vi "Actual Record Length.vi"(8 "error in (no error)":errorcluster, 11 "CS++Scope":refnum<class "CS++Scope.lvclass">) -> (0 "error out":errorcluster, 2 "actual record length":i32 caption="actual record length (samples)", 3 "CS++Scope out":refnum<class "CS++Scope.lvclass">)   [LabVIEW 2013, in "CS++Scope.lvlib" / "CS++Scope.lvclass"]
doc: "This VI returns the actual number of points the oscilloscope acquires for each channel. After you configure the oscilloscope for an acquisition, call this VI to determine the size of the waveforms that the oscilloscope acquires. The value is greater than or equal to the minimum number of points you specify in the IviScope Configure Acquisition Record VI. \nYou can use this value as the Waveform Size parameter of the IviScope Read Waveform and IviScope Fetch Waveform VIs."
uses:
  CS++Scope.lvclass
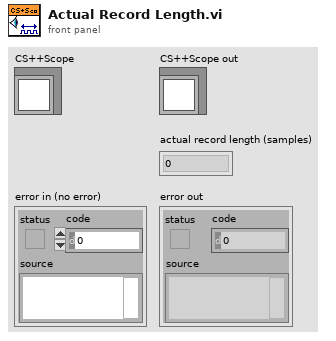
[diagram p1: front panel]
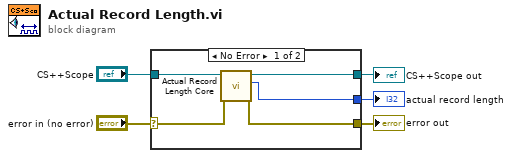
[diagram p0: block diagram]
diagram:
  n1 = case shown="No Error" "error in (no error)" {
    selector: "error in (no error)" -> [w8 w12]
    tunnel: [w7 w12] -> w4
    tunnel: [w9 w11] -> w2
    tunnel: "CS++Scope" -> [w10 w11]
    tunnel: [w6 _] -> w1
    frame No Error {
      n2 = call-dynamic "Actual Record Length Core.vi"("error in (no error)"=w8, "CS++Scope"=w10) -> ("error out"=w7:errorcluster, "actual record length"=w6:i32, "CS++Scope out"=w9:refnum<class "CS++Scope.lvclass">)  [unwired: 7 in]
    }
    frame Error {
    }
  }
  "error out" <- w4
  "actual record length" <- w1
  "CS++Scope out" <- w2
